vi "AddProjectConditionalDeactivationValuesByKeys.vi"(8 "Fehler (Eingang, kein Fehler)":errorcluster, 10 "CondDeact":cluster{"Keys":string[], "Values":string[]}, 11 "Set":cluster{"Keys":string[], "Values":string[]}) -> (0 "Fehler (Ausgang)":errorcluster, 2 "CondDeact out":cluster{"Keys":string[], "Values":string[]})   [LabVIEW 2015, in "ConditionalDeactivation.lvlib"]
uses:
  ConditionalDeactivation.lvlib
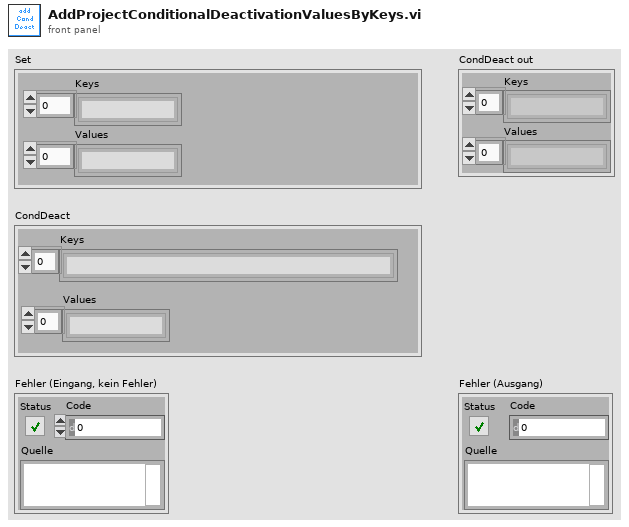
[diagram p1: front panel]
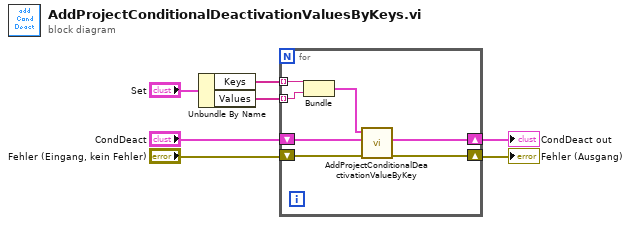
[diagram p0: block diagram]
diagram:
  n1 = Unbundle By Name("Set") -> ("Keys"=w3:string[], "Values"=w2:string[])
  n2 = for {
    shift-right: [w13] -> w5
    shift-left: "Fehler (Eingang, kein Fehler)" -> [w14]
    tunnel: w3 -> [w11] mode=indexing
    tunnel: w2 -> [w10] mode=indexing
    shift-right: [w8] -> w1
    shift-left: "CondDeact" -> [w12]
    n3 = Bundle("Key"=w11, "Value"=w10) -> (w9:cluster{"Key":string, "Value":string})  [unwired: 1 in]
    n4 = call "AddProjectConditionalDeactivationValueByKey.vi"("Fehler (Eingang, kein Fehler)"=w14, "CondDeact"=w12, "Set"=w9) -> ("Fehler (Ausgang)"=w13:errorcluster, "Ausgangs-Cluster"=w8:cluster{string[], string[]})  [unwired: 7 in]
  }
  "Fehler (Ausgang)" <- w5
  "CondDeact out" <- w1
